vi "CSU22 Test Panel.vi"() -> ()   [LabVIEW 2020]
uses:
  <vilib>/Instr/_visa.llb/VISA Configure Serial Port (Instr).vi
panel:
  out "Boolean array":bool[][](array[boolean])
  out "Disk Speed (RPM)":i32
  out "ND Filter Out?":bool
  out "Shutter Open?":bool
  out "Command History":string
  out "Success?":bool
  out "Waiting":bool
  out "Error":errorcluster
  in  "Quit":bool
  in  "Send Command":bool
  out "Reply":string
  in  "Command":string
  in  "COM Port":refnum<visa-resource-name>
  # "iz0 - initialize to factory default settings\niz1 - initialize to USER default settings (not sure what this means)\n\nsh0 - open the shutter\nsh1 - close the shutter\n\nla0 - move all filters back one step\nla1 - move all filters forward one step\n\nnd0 - add an ND filter with 10% transmission to the light path (I think)\nnd1 - no ND filter (I think)\n\nmsXXXX - disk speed with range between 1500 and 5000 RPM\n\nedbX1X2X3 - set specific filter positions with X1, X2, and X3 between 0 and 3. Zero means keep the current position.\nX1 must equal X3 to ensure the excitation and barrier filters always match (for safety).\n\nrsm - Get the current disk speed\nrsn - get ND filter position, result is in the 3rd bit, shutter position is in other bit (2?)\nrsf - get filter set position, filter status info is in bits 1 and 2\n\n:A means the command is done\n:N means the command was not understood"
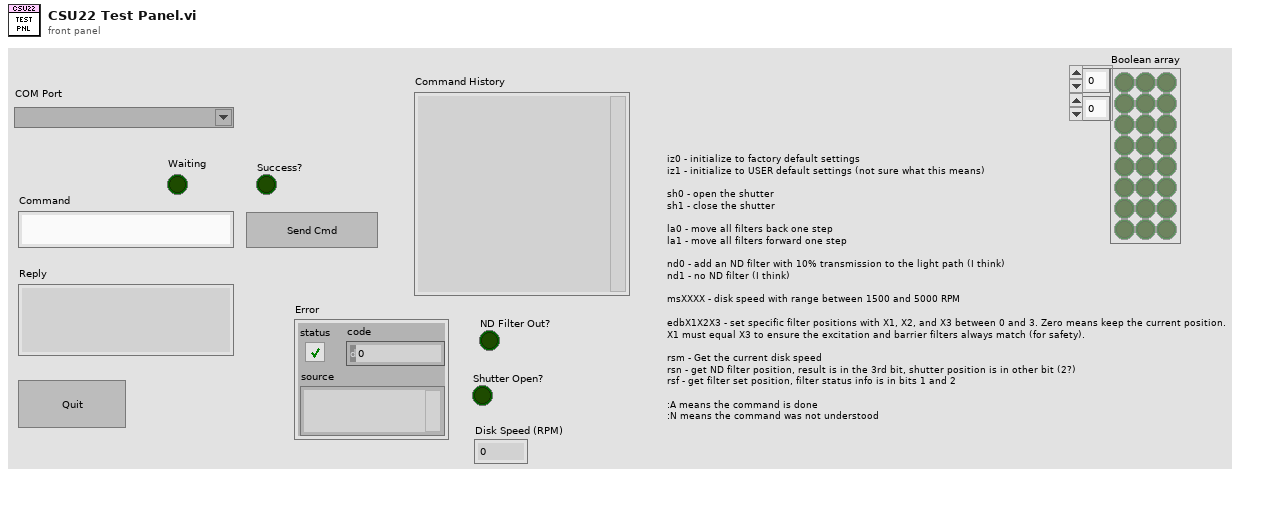
[diagram p1: front panel]
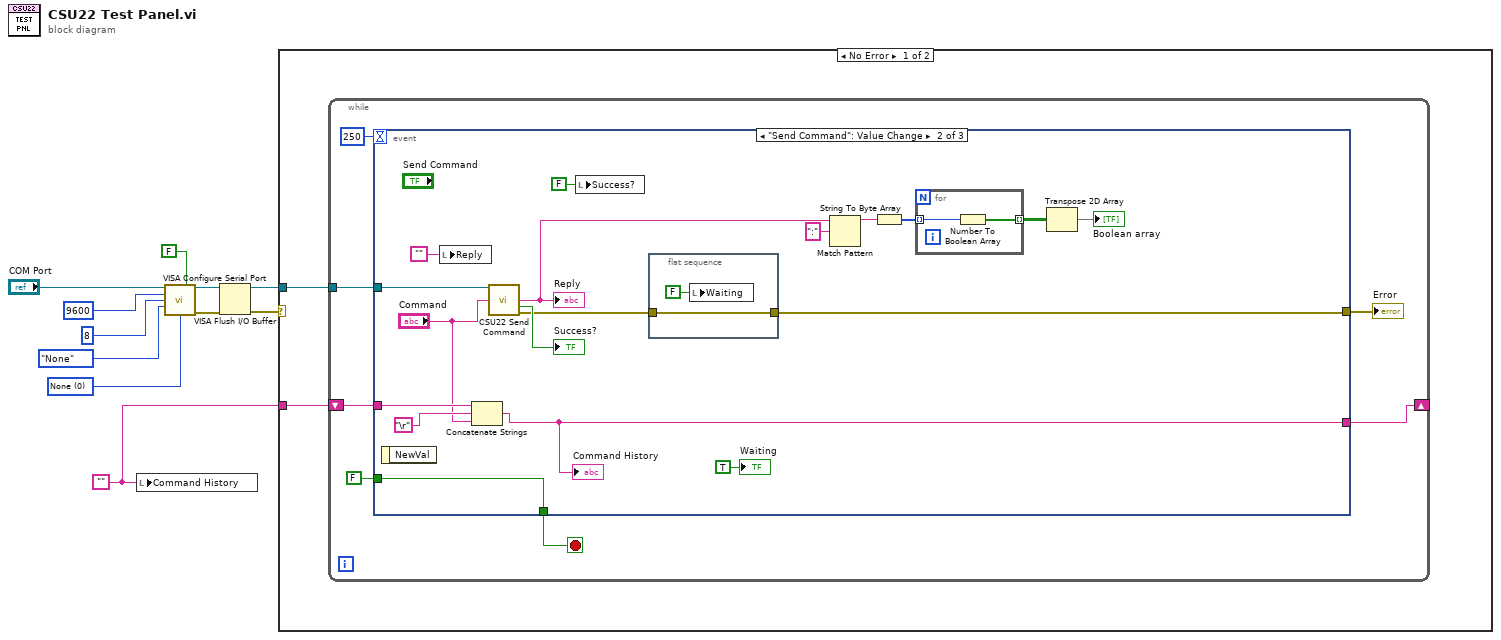
[diagram p0: block diagram]
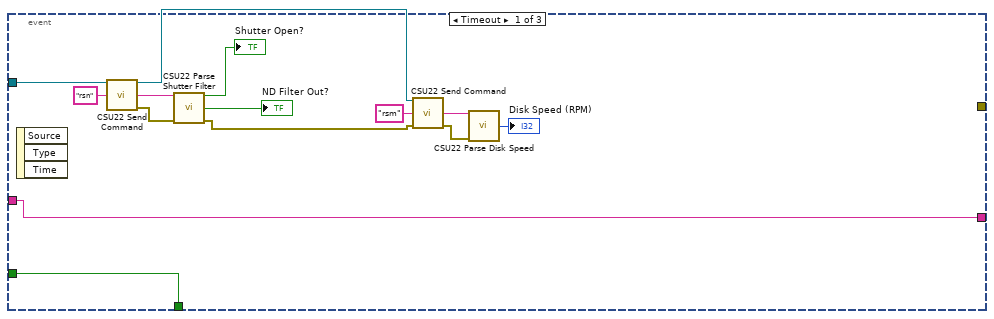
[diagram p2: hidden frame]
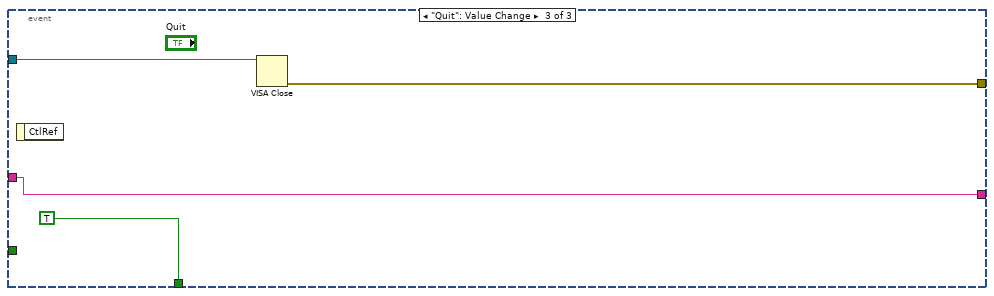
[diagram p3: hidden frame]
diagram:
  w1 = ""
  w6 = u16 0 items=["None", "XON/XOFF", "RTS/CTS", "XON/XOFF & RTS/CTS", "DTR/DSR", "XON/XOFF & DTR/DSR"] ("flow control (0:none)")
  n1 = local write "Command History"(w1) -> ()
  n2 = call-poly "VISA Configure Serial Port"("VISA resource name"="COM Port", "Enable Termination\nChar (T)"=FALSE ("Enable Termination\nChar (T)"), "baud rate (9600)"=u32 9600, "data bits (8)"=u16 8, "parity (0:none)"=enum16{"None", "Odd", "Even", "Mark", "Space"}."None", "flow control (0:none)"=w6) -> ("VISA resource name out"=w5:refnum<visa-resource-name>, "error out"=w4:errorcluster)  [unwired: 8 in]
  n3 = VISA Flush I/O Buffer(VISA resource name=w5, error in (no error)=w4) -> (VISA resource name out=w2:refnum<visa-resource-name>, error out=w3:errorcluster)  [unwired: 1 in]
  n4 = case shown="No Error" w3 {
    tunnel: w2 -> [w13 _]
    tunnel: w1 -> [w12 _]
    frame No Error {
      n5 = while {
        tunnel: w13 -> [w18]
        shift-right: [w15] -> _
        shift-left: w12 -> [w16]
        stop <- w19 stop-if-true
        n6 = event shown="[1] \"Send Command\": Value Change" {
          selector: _ -> [_ _ _]
          dyn-events: _ -> [_ _ _]
          timeout: 250 -> [_ _ _]
          tunnel: [w34 w52 TRUE] -> w19
          tunnel: FALSE -> [w34 w52 _]
          tunnel: w18 -> [w32 w49 w59]
          tunnel: [_ w48 w58] -> w17
          tunnel: w16 -> [w33 w45 w57]
          tunnel: [w33 w42 w57] -> w15
          event Timeout {
            n7 = event-data() -> ()  [unwired: 1 in, 3 out]
            n8 = call "CSU22 Send Command.vi"("VISA Ref"=w32, "Command"="rsn") -> ("VISA Ref Dup"=w24:refnum<visa-resource-name>, "Reply"=w30:string, "Error Out"=w29:errorcluster)  [unwired: 10 in, 1 out]
            n9 = call "CSU22 Parse Shutter Filter.vi"("Reply String"=w30, "Error In"=w29) -> ("Shutter Open?"=→"Shutter Open?":bool, "ND Filter Out?"=→"ND Filter Out?":bool, "Error Out"=w25:errorcluster)  [unwired: 11 in]
            n10 = call "CSU22 Send Command.vi"("VISA Ref"=w24, "Command"="rsm", "Error In"=w25) -> ("Reply"=w23:string, "Error Out"=w22:errorcluster)  [unwired: 9 in, 2 out]
            n11 = call "CSU22 Parse Disk Speed.vi"("Reply String"=w23, "Error In"=w22) -> ("Speed (RPM)"=→"Disk Speed (RPM)":i32)  [unwired: 12 in, 1 out]
          }
          event "Send Command": Value Change {
            n12 = event-data() -> ()  [unwired: 1 in, 1 out]
            n13 = local write "Reply"("") -> ()
            n14 = Concatenate Strings(w45, "\r", "Command") -> (w42:string)
            "Command History" <- w42
            n15 = call "CSU22 Send Command.vi"("VISA Ref"=w49, "Command"="Command") -> ("Reply"=w38:string, "Success?"=→"Success?":bool, "Error Out"=w41:errorcluster)  [unwired: 10 in, 1 out]
            "Reply" <- w38
            n16 = local write "Success?"(FALSE ("Success?")) -> ()
            n17 = flat-sequence {
              tunnel: w41 -> [w56]
              tunnel: [w56] -> w48
              frame #0 {
                n18 = local write "Waiting"(FALSE ("Waiting")) -> ()
              }
            }
            n19 = Match Pattern(string=w38, regular expression=":") -> (before substring=w39:string)  [unwired: 1 in, 3 out]
            n20 = String To Byte Array(string=w39) -> (unsigned byte array=w37:u8[])
            n21 = for {
              tunnel: w37 -> [w54] mode=indexing
              tunnel: [w53] -> w36 mode=indexing
              n22 = Number To Boolean Array(number=w54) -> (Boolean array=w53:bool[])
            }
            n23 = Transpose 2D Array(2D array=w36) -> (transposed array=→"Boolean array":bool[][])
            "Waiting" <- TRUE ("Waiting")
          }
          event "Quit": Value Change {
            n24 = event-data() -> ()  [unwired: 1 in, 1 out]
            n25 = VISA Close(VISA resource name=w59) -> (error out=w58:errorcluster)  [unwired: 1 in]
          }
        }
        "Error" <- w17
      }
    }
    frame Error {
    }
  }
